vi "String to Complex Number (CXT 1D Array).vi"(2 "use system decimal point (T)":bool=TRUE, 3 "default (0 CDB)":cxt, 4 "offset":i32, 5 "strings[]":string[](array[string])) -> (0 "numbers[]":cxt[](array[numeric]), 1 "offsets past number[]":i32[](array[numeric]))   [LabVIEW 2018, in "Numeric Data Type.lvclass"]
doc: "<b> </b> <b> </b>\n©2013, Q Software Innovations, LLC.\n\nWritten in National Instruments LabVIEW™ 2013.\n\nAuthored by Quentin Alldredge\nQ@qsoftwareinnovations.com\nwww.qsoftwareinnovations.com\n\nAll rights reserved."
uses:
  Numeric Data Type.lvclass
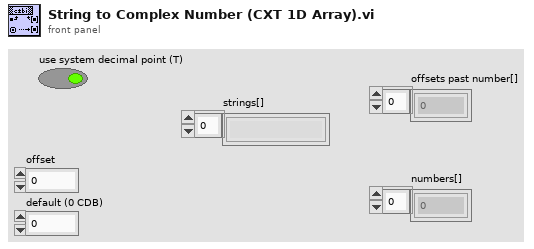
[diagram p1: front panel]
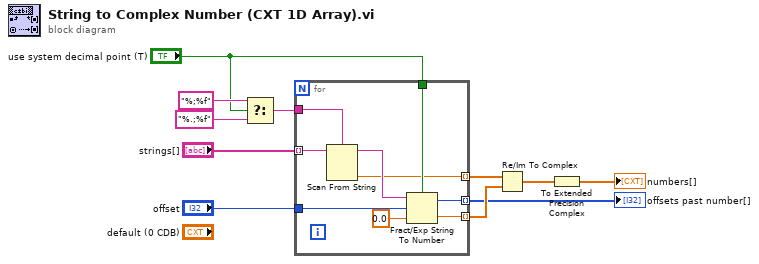
[diagram p0: block diagram]
diagram:
  n1 = Select(t="%;%f", s="use system decimal point (T)", f="%.;%f") -> (s? t:f=w9:string)
  n2 = for {
    tunnel: w9 -> [w20]
    tunnel: "use system decimal point (T)" -> [w18]
    tunnel: [w17] -> w7 mode=indexing
    tunnel: [w16] -> w6 mode=indexing
    tunnel: "offset" -> [w14]
    tunnel: [w13] -> w2 mode=indexing
    tunnel: "strings[]" -> [w12] mode=indexing
    n3 = Scan From String(format string=w20, input string=w12) -> (remaining string=w19:string, output 1=w17:dbl)  [unwired: 3 in, 2 out]
    n4 = Fract/Exp String To Number(use system decimal point (T)=w18, string=w19, offset=w14, default (0 dbl)=0.0 ("default (0 DBL)")) -> (offset past number=w13:i32, number=w16:dbl)
  }
  "offsets past number[]" <- w2
  n5 = Re/Im To Complex(1:w6, 2:w7) -> (0:w3:cdb[])
  n6 = To Extended Precision Complex(1:w3) -> (0:→"numbers[]":cxt[])
